vi "10HzLogLoop_HDF5_20210610.vi"(8 "error in":errorcluster, 11 "queue in":refnum<queue>) -> (0 "error out":errorcluster)   [LabVIEW 2018]
uses:
  Controls/Enums/10Hz_Loop_Enum.ctl
  Controls/Clusts/10Hz_Loop_Clust.ctl
  Controls/Clusts/HDF5_10HzRefs.ctl
  <vilib>/addons/h5labview2/base/hid_t.ctl
  Controls/Clusts/10Hz_Data.ctl
  Controls/Enums/TargetNumber.ctl
  <vilib>/addons/h5labview2/file/H5Fmode.ctl
  <vilib>/addons/h5labview2/base/lib_path.vi
  <vilib>/addons/h5labview2/base/H5Equery.vi
  <vilib>/addons/h5labview2/dataset/H5Dwrite.llb/H5Dwrite.xnode
  <vilib>/addons/h5labview2/file/H5F.lvlib
  <vilib>/addons/h5labview2/dataset/H5D.lvlib
  <vilib>/addons/h5labview2/space/H5S.lvlib
panel:
  out "Numeric":i32
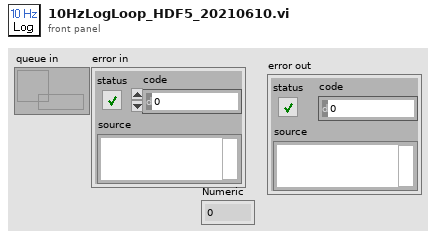
[diagram p1: front panel]
types:
  T1 = typedef "10Hz_Loop_Clust.ctl" = cluster{"Refs":T2, "DateString":string, "StartTime":timestamp, "Data":T4, "LogFolder":path}
  T2 = typedef "HDF5_10HzRefs.ctl" = cluster{"72Co_dset":T3, "84Co_dset":T3, "FileRef":T3}
  T3 = typedef "hid_t.ctl" = i32
  T4 = typedef "10Hz_Data.ctl" = cluster{"PeakVal":dbl[], "Channel":T5, "TimeStamp":timestamp}
  T5 = typedef "TargetNumber.ctl" = enum16{"1", "2", "3", "4"}
  T6 = typedef "H5F.lvlib/H5Fmode.ctl" = enum16{"read-only", "read-write", "overwrite", "create new", "open or create"}
  T7 = typedef "10Hz_Loop_Enum.ctl" = enum16{"10Hz_Init", "10Hz_Cfg", "10Hz_NewData", "10Hz_Write", "10Hz_Stop"}
  T8 = cluster{"72Co_dset":i32, "84Co_dset":i32, "FileRef":i32}
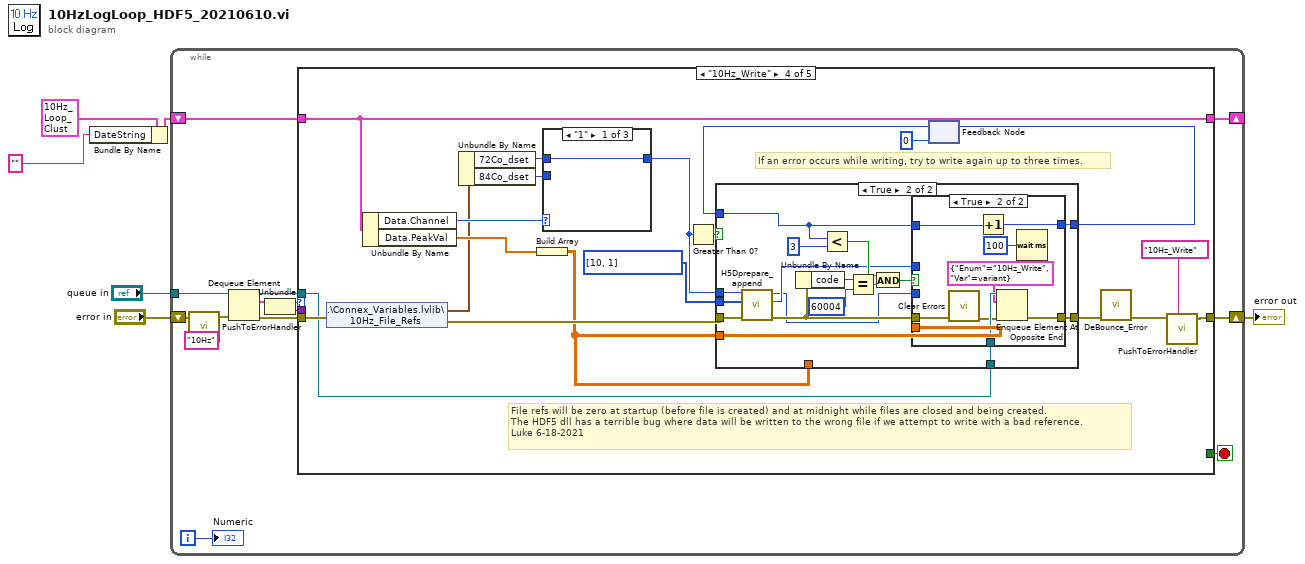
[diagram p0: block diagram]
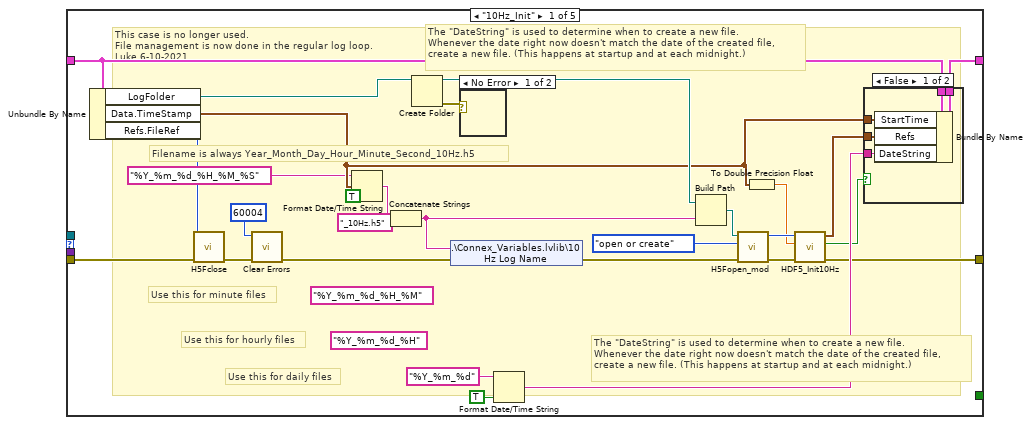
[diagram p2: hidden frame]
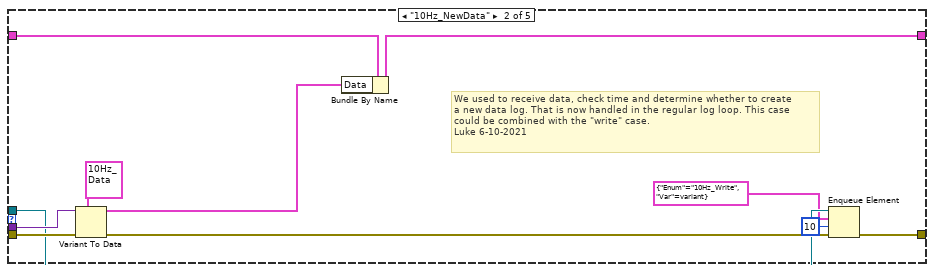
[diagram p5: hidden frame]
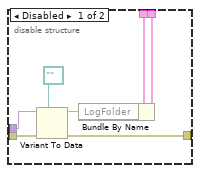
[diagram p7: hidden frame]
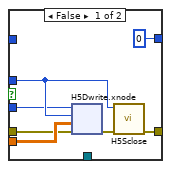
[diagram p9: hidden frame]
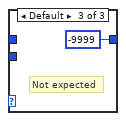
[diagram p11: hidden frame]
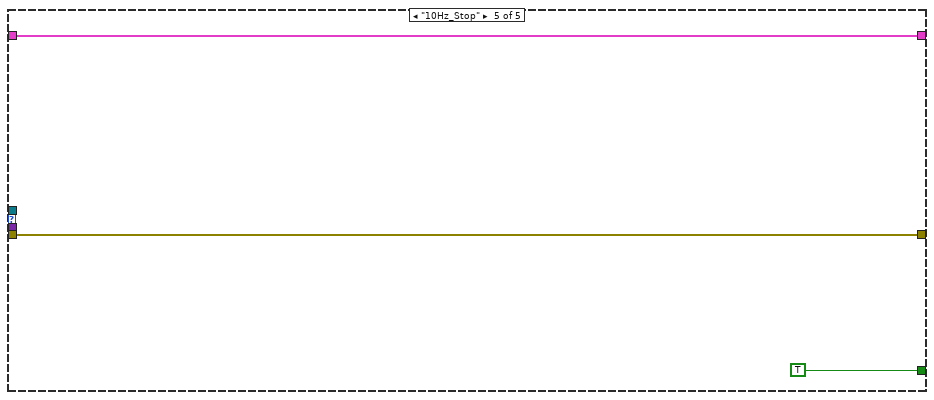
[diagram p12: hidden frame]
diagram:
  n1 = Bundle By Name(cluster=T1 {"Refs"={"72Co_dset"=0, "84Co_dset"=0, "FileRef"=0}, "DateString"="", "StartTime"=timestamp(0 s since 1904-01-01), "Data"={"PeakVal"=[], "Channel"=enum."4", "TimeStamp"=timestamp(0 s since 1904-01-01)}, "LogFolder"=path "C:/"}, "DateString"="") -> (w2:T1)
  n2 = while {
    tunnel: "queue in" -> [w7]
    shift-right: [w15] -> w3
    shift-left: "error in" -> [w14]
    shift-right: [w11] -> _
    shift-left: w2 -> [w12]
    i -> [w8]
    stop <- w9 stop-if-true
    n3 = call "PushToErrorHandler.vi"("ErrorIn"=w14, "ErrorLocation"="10Hz") -> ("ErrorOut"=w17:errorcluster)  [unwired: 5 in]
    n4 = Dequeue Element(queue=w7, error in (no error)=w17) -> (queue out=w10:refnum<queue>, element=w20:cluster{"Enum":T7, "Var":variant}, error out=w16:errorcluster)  [unwired: 1 in, 1 out]
    n5 = Unbundle(w20) -> ("Enum"=w19:T7, "Var"=w18:variant)
    n6 = case shown="\"10Hz_Write\"" w19 {
      tunnel: w18 -> [_ w64 w68 _ _]
      tunnel: w16 -> [w30 w65 w69 w91 w158]
      tunnel: [w36 w59 w66 w84 w158] -> w15
      tunnel: w12 -> [w34 w57 w70 w99 w157]
      tunnel: [w35 w61 w67 w99 w157] -> w11
      tunnel: w10 -> [_ w58 _ w88 _]
      tunnel: [_ _ _ _ TRUE] -> w9
      frame "10Hz_Init" {
        (unwired) "%Y_%m_%d_%H_%M" ("time format string (%c)")
        (unwired) "%Y_%m_%d_%H" ("time format string (%c)")
        # "This case is no longer used.\nFile management is now done in the regular log loop.\nLuke 6-10-2021"
        # "Use this for minute files"
        # "Use this for hourly files"
        # "The \"DateString\" is used to determine when to create a new file.\nWhenever the date right now doesn't match the date of the created file,\ncreate a new file. (This happens at startup and at each midnight.)"
        # "Use this for daily files"
        # "Filename is always Year_Month_Day_Hour_Minute_Second_10Hz.h5"
        # "The \"DateString\" is used to determine when to create a new file.\nWhenever the date right now doesn't match the date of the created file,\ncreate a new file. (This happens at startup and at each midnight.)"
        n7 = Unbundle By Name(w34) -> ("LogFolder"=w23:path, "Data.TimeStamp"=w25:timestamp, "Refs.FileRef"=w32:T3)
        n8 = call <vilib>:"H5Fclose.vi"("error in (no error)"=w30, "ref"=w32) -> ("error out"=w33:errorcluster)  [unwired: 9 in]
        n9 = call <vilib>:"Clear Errors.vi"("error in (no error)"=w33, "specific error code to clear (0: all)"=60004) -> ("error out"=w28:errorcluster)  [unwired: 4 in, 1 out]
        n10 = Format Date/Time String(time format string (%c)="%Y_%m_%d_%H_%M_%S", seconds (now)=w25, UTC format=TRUE) -> (date/time string=w46:string)
        n11 = Concatenate Strings(w46, "_10Hz.h5" ("string")) -> (w29:string)
        n12 = Create Folder(path (use dialog)=w23) -> (created path=w48:path, error out=w47:errorcluster)  [unwired: 2 in, 1 out]
        n13 = shared-variable ".\\Connex_Variables.lvlib\\10 Hz Log Name"(w29, error in=w28) -> (error out=w27:errorcluster)
        n14 = case shown="No Error" w47 {
          frame No Error {
          }
          frame Error {
          }
        }
        n15 = Format Date/Time String(time format string (%c)="%Y_%m_%d", UTC format=TRUE) -> (date/time string=w37:string)  [unwired: 1 in]
        n16 = Build Path(base path=w48, name or relative path=w29) -> (appended path=w43:path)
        n17 = call "H5Fopen_mod.vi"("error in (no error)"=w27, "mode (read-only)"=H5Fmode."open or create", "path"=w43) -> ("error out"=w41:errorcluster, "ref out"=w42:T3)  [unwired: 6 in, 1 out]
        n18 = To Double Precision Float(number=w25) -> (double precision float=w26:dbl)
        n19 = call "HDF5_Init10Hz.vi"("error in (no error)"=w41, "TimeStamp"=w26, "FileRef"=w42) -> ("error out"=w36:errorcluster, "Invalid"=w22:bool, "10HzRef"=w39:T2)  [unwired: 6 in]
        n20 = case shown="False" w22 {
          tunnel: w39 -> [w53 _]
          tunnel: w37 -> [w52 _]
          tunnel: [w51 w54] -> w35
          tunnel: w34 -> [w50 w54]
          tunnel: w25 -> [w49 _]
          frame False {
            n21 = Bundle By Name(cluster=w50, "StartTime"=w49, "Refs"=w53, "DateString"=w52) -> (w51:T1)
          }
          frame True {
          }
        }
      }
      frame "10Hz_NewData" {
        # "We used to receive data, check time and determine whether to create\na new data log. That is now handled in the regular log loop. This case\ncould be combined with the \"write\" case.\nLuke 6-10-2021"
        n22 = Variant To Data(error in=w65, type=T4 {"PeakVal"=[], "Channel"=enum."4", "TimeStamp"=timestamp(0 s since 1904-01-01)} ("Data"), Variant=w64) -> (data=w62:T4, error out=w60:errorcluster)
        n23 = Bundle By Name(cluster=w57, "Data"=w62) -> (w61:T1)
        n24 = Enqueue Element(queue=w58, element=cluster{"Enum":T7, "Var":variant} {"Enum"=enum."10Hz_Write", "Var"=variant}, timeout in ms (-1)=10, error in (no error)=w60) -> (error out=w59:errorcluster)  [unwired: 2 out]
      }
      frame "10Hz_Cfg" {
        # "This case is no longer used.\nFile management is now handled in the regular log loop."
        n25 = disable-structure shown="Enabled" {
          disable-tunnel: w70 -> [w77 w79]
          disable-tunnel: w69 -> [w76 w78]
          disable-tunnel: w68 -> [w75 _]
          disable-tunnel: [w74 w79] -> w67
          disable-tunnel: [w73 w78] -> w66
          frame Disabled {
            n26 = Variant To Data(error in=w76, type=path "" ("LogFolder"), Variant=w75) -> (data=w71:path, error out=w73:errorcluster)
            n27 = Bundle By Name(cluster=w77, "LogFolder"=w71) -> (w74:T1)
          }
          frame Enabled {
          }
        }
      }
      frame "10Hz_Write" {
        # "File refs will be zero at startup (before file is created) and at midnight while files are closed and being created.\nThe HDF5 dll has a terrible bug where data will be written to the wrong file if we attempt to write with a bad reference.\nLuke 6-18-2021"
        # "If an error occurs while writing, try to write again up to three times."
        n28 = shared-variable ".\\Connex_Variables.lvlib\\10Hz_File_Refs"(error in=w91) -> (w95:T8, error out=w92:errorcluster)
        n29 = Unbundle By Name(w99) -> ("Data.Channel"=w96:T5, "Data.PeakVal"=w97:dbl[])
        n30 = Unbundle By Name(w95) -> ("72Co_dset"=w94:i32, "84Co_dset"=w93:i32)
        n31 = Build Array(w97) -> (w82:dbl[][])
        n32 = case shown="\"1\"" w96 {
          tunnel: w94 -> [w153 _ _]
          tunnel: w93 -> [_ w154 _]
          tunnel: [w153 w154 T3 -9999 ("84Co_dset")] -> w90
          frame "1" {
          }
          frame "3" {
          }
          frame Default {
            # "Not expected"
          }
        }
        n33 = Greater Than 0?(x=w90) -> (x > 0?=w89:bool)
        n34 = feedback #1(0) -> (w85:i32)
        n35 = case shown="True" w89 {
          tunnel: w82 -> [_ _]
          tunnel: u64[] [10, 1] ("append dims") -> [_ w118]
          tunnel: [w101 w115] -> w81
          tunnel: w92 -> [w101 w106]
          tunnel: w90 -> [_ w107]
          tunnel: w88 -> [_ w117]
          tunnel: [w100 w116] -> w86
          tunnel: w85 -> [w100 w110]
          tunnel: w82 -> [_ w103]
          frame False {
            # "If file hasn't been configured, \ndon't try to write.\nUninitialized = 0\nFailed initialize = -1"
          }
          frame True {
            n36 = call <vilib>:"H5Dprepare_append.vi"("error in (no error)"=w106, "append dims"=w118, "dset in"=w107) -> ("error out"=w105:errorcluster, "space out"=w104:T3, "dset out"=w102:T3)  [unwired: 5 in, 1 out]
            n37 = Unbundle By Name(w105) -> ("code"=w114:i32)
            n38 = Less?(x=w110, y=3) -> (x < y?=w109:bool)
            n39 = Equal?(x=w114, y=60004 ("x")) -> (x = y?=w113:bool)
            n40 = And(x=w109, y=w113) -> (x .and. y?=w111:bool)
            n41 = case shown="True" w111 {
              tunnel: [w119 w152] -> w115
              tunnel: w117 -> [_ w151]
              tunnel: w105 -> [w121 w149]
              tunnel: [0 w147] -> w116
              tunnel: w110 -> [_ w146]
              tunnel: w104 -> [w123 _]
              tunnel: w103 -> [w124 _]
              tunnel: w102 -> [w122 _]
              frame False {
                n42 = xnode "H5Dwrite.xnode"("error in (no error)"=w121, "data"=w124, "file space"=w123, "ref in"=w122) -> ("error out"=w120:errorcluster)  [unwired: 3 in, 2 out]
                n43 = call <vilib>:"H5Sclose.vi"("error in (no error)"=w120, "space in"=w123) -> ("error out"=w119:errorcluster)  [unwired: 9 in]
              }
              frame True {
                n44 = call <vilib>:"Clear Errors.vi"("error in (no error)"=w149) -> ("error out"=w148:errorcluster)  [unwired: 5 in, 1 out]
                n45 = Increment(x=w146) -> (x+1=w147:i32)
                n46 = Enqueue Element At Opposite End(queue=w151, element=cluster{"Enum":T7, "Var":variant} {"Enum"=enum."10Hz_Write", "Var"=variant}, error in (no error)=w148) -> (error out=w152:errorcluster)  [unwired: 1 in, 2 out]
                n47 = Wait (ms)(milliseconds to wait=u32 100) -> ()  [unwired: 1 out]
              }
            }
          }
        }
        n48 = feedback-in #1(w86) -> ()
        n49 = call "DeBounce_Error.vi"("error in (no error)"=w81) -> ("error out"=w80:errorcluster)  [unwired: 10 in]
        n50 = call "PushToErrorHandler.vi"("ErrorIn"=w80, "ErrorLocation"="10Hz_Write") -> ("ErrorOut"=w84:errorcluster)  [unwired: 5 in]
      }
      frame "10Hz_Stop" {
      }
    }
    "Numeric" <- w8
  }
  "error out" <- w3
